vi "Read Data Model.vi"(8 "error in (no error)":errorcluster, 11 "Modbus slave in":refnum<class "Modbus Slave.lvclass">) -> (0 "error out":errorcluster, 2 "device data model":refnum<class "Device Data Model.lvclass">, 3 "Modbus slave out":refnum<class "Modbus Slave.lvclass">)   [LabVIEW 2021, in "Modbus Slave.lvclass"]
doc: "This VI is an accessor for the <B>data model</B> stored in the Modbus master instance. This accessor can be used as a property node. This model defines how the slave stores data and reacts to functions and data sent by a Modbus master."
uses:
  Modbus Slave.lvclass
  Data Model/Device Data Model.lvclass
  Modbus Slave.lvclass/Modbus Slave.ctl
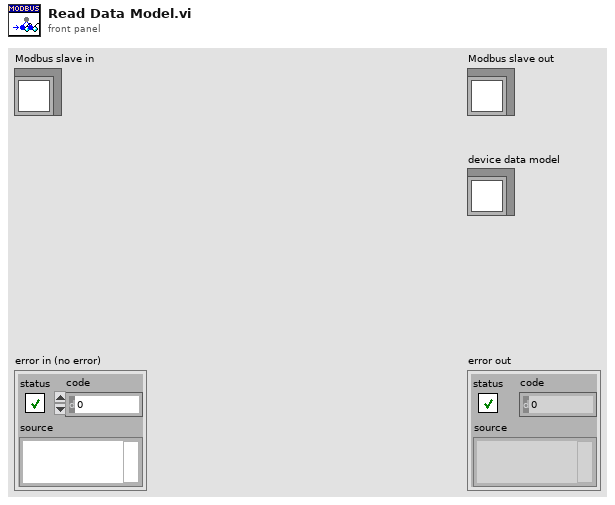
[diagram p1: front panel]
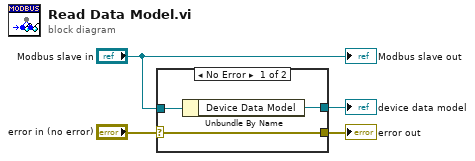
[diagram p0: block diagram]
diagram:
  n1 = case shown="No Error" "error in (no error)" {
    selector: "error in (no error)" -> [w5 w8]
    tunnel: "Modbus slave in" -> [w7 _]
    tunnel: [w6 _] -> w3
    tunnel: [w5 w8] -> w1
    frame No Error {
      n2 = Unbundle By Name(w7) -> ("Device Data Model"=w6:refnum<class "Device Data Model.lvclass">)
    }
    frame Error {
    }
  }
  "error out" <- w1
  "device data model" <- w3
  "Modbus slave out" <- "Modbus slave in"
